vi "RobotSimulatorAvanced.vi"() -> ()   [LabVIEW 2020]
uses:
  530416c0-6674-4c07-96e2-8651c6c7ac9e.vi
  e8d99151-f8ba-459a-ac77-b5781a9d7d4b.vi
  <vilib>/Utility/inputDevices.llb/joystickAcquire.vi
  <vilib>/Utility/inputDevices.llb/closeJoystick.vi
panel:
  out "SorN":i32
  out "Ativ.":bool
  out "?":dbl(knob) scale=-100.0..100.0 scale format="%#.1f"
  out "Trás Esq.":bool
  out "Frente Dir.":bool
  out "Trás Dir.":bool
  out "Frente Esq.":bool
  out "joystick info":T1(array[cluster])
  out "direction info":T2
  out "button info":T3
  out "axis info":T4
  # "Velocidade"
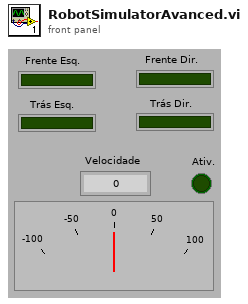
[diagram p1: front panel]
types:
  T1 = cluster{"axes total":u32, "buttons total":u32, "pov total":u32, "device name":string}[]
  T2 = cluster{"pov 1":i32, "pov 2":i32, "pov 3":i32, "pov 4":i32}
  T3 = cluster{"button 1":bool, "button 2":bool, "button 3":bool, "button 4":bool, "button 5":bool, "button 6":bool, "button 7":bool, "button 8":bool, "button 9":bool, "button 10":bool, "button 11":bool, "button 12":bool, "button 13":bool, "button 14":bool, "button 15":bool, "button 16":bool, "button 17":bool, "button 18":bool, "button 19":bool, "button 20":bool, "button 21":bool, "button 22":bool, "button 23":bool, "button 24":bool, "button 25":bool, "button 26":bool, "button 27":bool, "button 28":bool, "button 29":bool, "button 30":bool, "button 31":bool, "button 32":bool}
  T4 = cluster{"X axis":i32, "Y axis":i32, "Z axis":i32, "X axis rotation":i32, "Y axis rotation":i32, "Z axis rotation":i32, "U axis":i32, "V axis":i32}
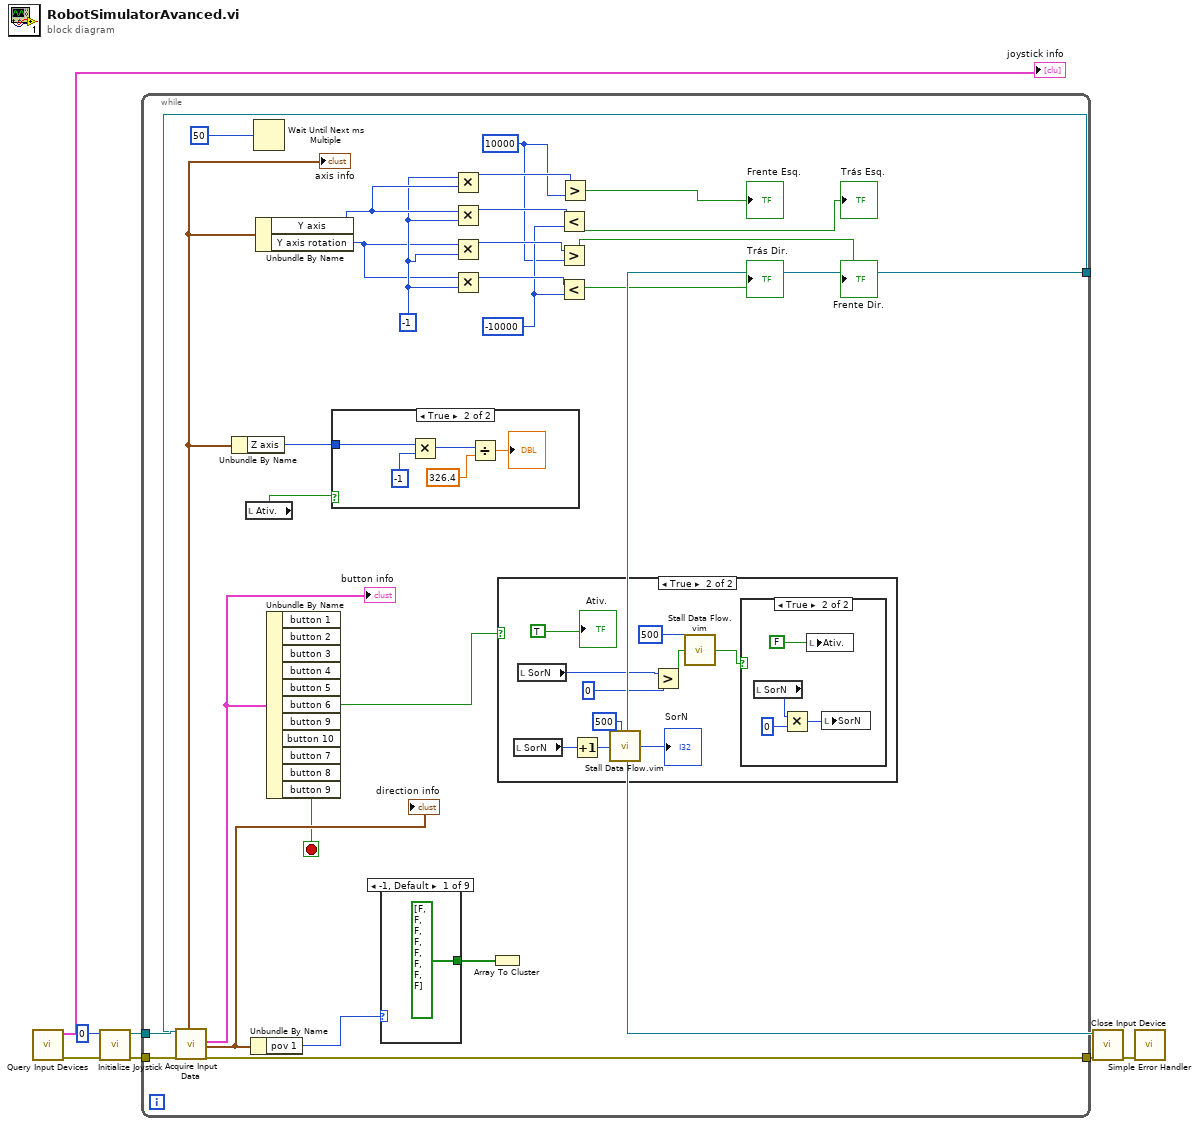
[diagram p0: block diagram]
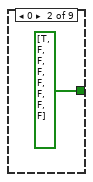
[diagram p5: hidden frame]
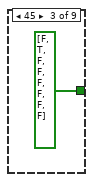
[diagram p6: hidden frame]
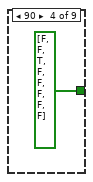
[diagram p7: hidden frame]
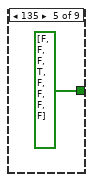
[diagram p8: hidden frame]
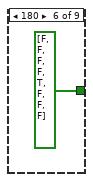
[diagram p9: hidden frame]
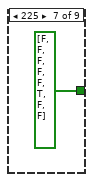
[diagram p10: hidden frame]
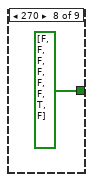
[diagram p11: hidden frame]
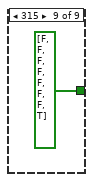
[diagram p12: hidden frame]
diagram:
  n1 = call <vilib>:"Query Input Devices.vi"() -> ("error out"=w2:errorcluster, "joystick info"=→"joystick info":T1)  [unwired: 1 in, 9 out]
  n2 = call <vilib>:"Initialize Joystick.vi"("error in (no error)"=w2, "device index"=0) -> ("error out"=w6:errorcluster, "device ID"=w7:refnum<k1>)  [unwired: 8 out]
  n3 = while {
    tunnel: w7 -> [w35]
    tunnel: w6 -> [w34]
    tunnel: [w33] -> w5
    tunnel: [w28] -> w4
    stop <- w27 stop-if-true
    w13 = 10000
    w14 = -10000
    w23 = -1
    n4 = call-poly <vilib>:"Acquire Input Data.vi"("device ID"=w35, "error in (no error)"=w34) -> ("device ID"=w33:refnum<k1>, "axis info"=w25:T4, "button info"=w32:T3, "direction info"=w31:T2, "error out"=w28:errorcluster)  [unwired: 13 out]
    "axis info" <- w25
    "button info" <- w32
    "direction info" <- w31
    n5 = Unbundle By Name(w25) -> ("Z axis"=w10:i32)
    n6 = local read "Ativ."() -> (w9:bool)
    n7 = Unbundle By Name(w31) -> ("pov 1"=w30:i32)
    n8 = Wait Until Next ms Multiple(millisecond multiple=u32 50) -> ()  [unwired: 1 out]
    n9 = Unbundle By Name(w25) -> ("Y axis"=w24:i32, "Y axis rotation"=w22:i32)
    n10 = Unbundle By Name(w32) -> ("button 6"=w11:bool, "button 7"=w27:bool)  [unwired: 9 out]
    n11 = case shown="True" w9 {
      tunnel: w10 -> [_ w36]
      frame False {
      }
      frame True {
        n12 = Multiply(x=w36, y=-1) -> (x*y=w40:i32)
        n13 = Divide(x=w40, y=326.4) -> (x/y=→"?":dbl)
      }
    }
    n14 = case shown="-1, Default" w30 {
      tunnel: [bool[] [FALSE, FALSE, FALSE, FALSE, FALSE, FALSE, FALSE, FALSE] ("Array") bool[] [TRUE, FALSE, FALSE, FALSE, FALSE, FALSE, FALSE, FALSE] ("Array") bool[] [FALSE, TRUE, FALSE, FALSE, FALSE, FALSE, FALSE, FALSE] ("Array") bool[] [FALSE, FALSE, TRUE, FALSE, FALSE, FALSE, FALSE, FALSE] ("Array") bool[] [FALSE, FALSE, FALSE, TRUE, FALSE, FALSE, FALSE, FALSE] ("Array") bool[] [FALSE, FALSE, FALSE, FALSE, TRUE, FALSE, FALSE, FALSE] ("Array") bool[] [FALSE, FALSE, FALSE, FALSE, FALSE, TRUE, FALSE, FALSE] ("Array") bool[] [FALSE, FALSE, FALSE, FALSE, FALSE, FALSE, TRUE, FALSE] ("Array") bool[] [FALSE, FALSE, FALSE, FALSE, FALSE, FALSE, FALSE, TRUE] ("Array")] -> w29
      frame -1, Default {
      }
      frame 0 {
      }
      frame 45 {
      }
      frame 90 {
      }
      frame 135 {
      }
      frame 180 {
      }
      frame 225 {
      }
      frame 270 {
      }
      frame 315 {
      }
    }
    n15 = Multiply(x=w23, y=w24) -> (x*y=w15:i32)
    n16 = Multiply(x=w24, y=w23) -> (x*y=w18:i32)
    n17 = Multiply(x=w22, y=w23) -> (x*y=w20:i32)
    n18 = Multiply(x=w22, y=w23) -> (x*y=w19:i32)
    n19 = Array To Cluster(array=w29) -> ()  [unwired: 1 out]
    n20 = case shown="True" w11 {
      frame False {
      }
      frame True {
        n21 = local read "SorN"() -> (w49:i32)
        n22 = local read "SorN"() -> (w42:i32)
        n23 = Increment(x=w49) -> (x+1=w48:i32)
        n24 = call "Stall Data Flow.vim"("value in"=w48, "milliseconds to wait"=u32 500) -> ("value out"=→"SorN":i32)  [unwired: 1 out]
        n25 = Greater?(x=w42, y=0) -> (0:w44:bool)
        n26 = call "Stall Data Flow.vim"("value in"=w44, "milliseconds to wait"=u32 500) -> ("value out"=w43:bool)  [unwired: 1 out]
        n27 = case shown="True" w43 {
          frame False {
          }
          frame True {
            n28 = local read "SorN"() -> (w53:i32)
            n29 = Multiply(x=w53, y=0) -> (x*y=w51:i32)
            n30 = local write "Ativ."(FALSE) -> ()
            n31 = local write "SorN"(w51) -> ()
          }
        }
        "Ativ." <- TRUE
      }
    }
    n32 = Less?(x=w18, y=w14) -> (x < y?=→"Trás Esq.":bool)
    n33 = Greater?(x=w20, y=w13) -> (0:→"Frente Dir.":bool)
    n34 = Less?(x=w19, y=w14) -> (x < y?=→"Trás Dir.":bool)
    n35 = Greater?(x=w15, y=w13) -> (0:→"Frente Esq.":bool)
  }
  n36 = call-poly <vilib>:"Close Input Device.vi"("error in (no error)"=w4, "device ID"=w5) -> ("error out"=w1:errorcluster)  [unwired: 8 out]
  n37 = call <vilib>:"Simple Error Handler.vi"("error in (no error)"=w1) -> ()  [unwired: 1 in, 8 out]
